vi "System_Conf.vi"() -> ()   [LabVIEW 2020]
uses:
  From/System_conf.ctl
panel:
  in  "system":T1
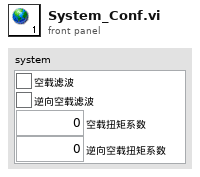
[diagram p1: front panel]
types:
  T1 = typedef "System_conf.ctl" = cluster{"空载滤波":bool, "逆向空载滤波":bool, "空载扭矩系数":dbl, "逆向空载扭矩系数":dbl}
diagram:
